vi "cal_inst.vi"() -> ()   [LabVIEW 2011]
panel:
  in  "Duration (0.00 seconds)":dbl format="%.2g"
  in  "Start Voltage (0.00 volts)":dbl format="%.2f"
  in  "End Voltage (0.00 volts)":dbl format="%.2g"
  out "Ramp In Progress":bool
  in  "Abort Ramp":bool
  in  "Current Limit (10.00 Amps)":dbl=10.0 format="%.2f"
  in  "Voltage Level (100.00 volts)":dbl=100.0 format="%.2f"
  in  "Voltage Range (150.00 volts)":dbl=150.0 format="%.2f"
  in  "Phase Name (\"\")":string
  in  "Frequency (60.00 Hz)":dbl=60.0 format="%.2f"
  in  "Frequency Range (600.00 Hz)":dbl=600.0 format="%.2f"
  in  "IVI Logical Name":refnum<k15>
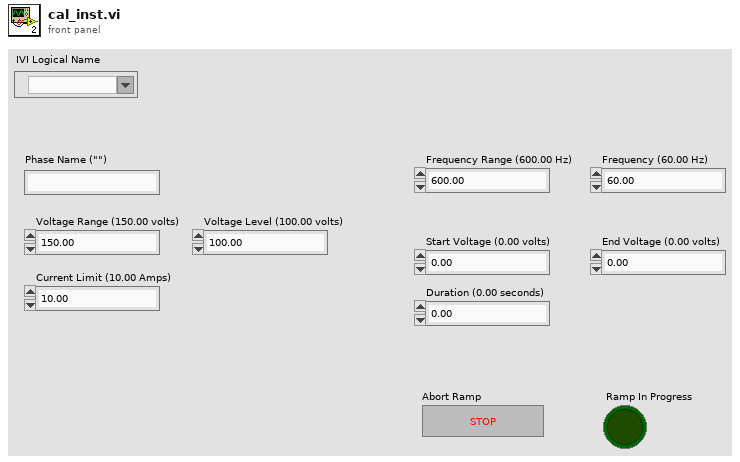
[diagram p1: front panel]
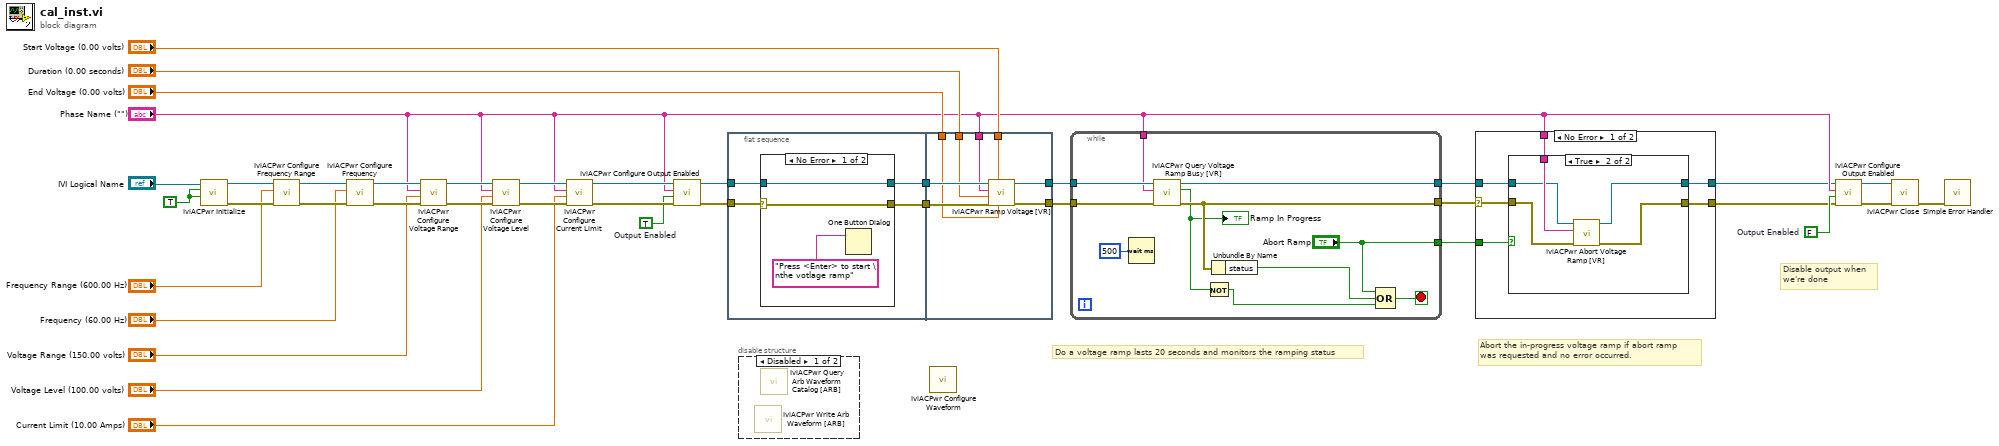
[diagram p0: block diagram]
diagram:
  w12 = FALSE  # Output Enabled
  w20 = TRUE  # Output Enabled
  w30 = TRUE ("id query (Yes)")
  # "Abort the in-progress voltage ramp if abort ramp\nwas requested and no error occurred."
  # "Disable output when\nwe're done"
  # "Do a voltage ramp lasts 20 seconds and monitors the ramping status"
  n1 = call <vilib>:"IviACPwr Initialize.vi"("reset device (Yes)"=w30, "id query (Yes)"=w30, "logical name (\"SampleACPwr\")"="IVI Logical Name") -> ("error out"=w36:errorcluster, "instrument handle out"=w37:refnum<k15>)  [unwired: 1 in, 6 out]
  n2 = call <vilib>:"IviACPwr Configure Frequency Range.vi"("error in (no error)"=w36, "Frequency Range"="Frequency Range (600.00 Hz)", "instrument handle"=w37) -> ("error out"=w34:errorcluster, "instrument handle out"=w35:refnum<k15>)  [unwired: 1 in, 6 out]
  n3 = call <vilib>:"IviACPwr Configure Frequency.vi"("error in (no error)"=w34, "Frequency"="Frequency (60.00 Hz)", "instrument handle"=w35) -> ("error out"=w32:errorcluster, "instrument handle out"=w33:refnum<k15>)  [unwired: 1 in, 6 out]
  n4 = call <vilib>:"IviACPwr Configure Voltage Range.vi"("error in (no error)"=w32, "Range"="Voltage Range (150.00 volts)", "Phase Name (\"\")"="Phase Name (\"\")", "instrument handle"=w33) -> ("error out"=w25:errorcluster, "instrument handle out"=w28:refnum<k15>)  [unwired: 6 out]
  n5 = call <vilib>:"IviACPwr Configure Voltage Level.vi"("error in (no error)"=w25, "Voltage Level"="Voltage Level (100.00 volts)", "Phase Name (\"\")"="Phase Name (\"\")", "instrument handle"=w28) -> ("error out"=w26:errorcluster, "instrument handle out"=w27:refnum<k15>)  [unwired: 6 out]
  n6 = call <vilib>:"IviACPwr Configure Current Limit.vi"("error in (no error)"=w26, "Limit"="Current Limit (10.00 Amps)", "Phase Name (\"\")"="Phase Name (\"\")", "instrument handle"=w27) -> ("error out"=w21:errorcluster, "instrument handle out"=w22:refnum<k15>)  [unwired: 6 out]
  n7 = call <vilib>:"IviACPwr Configure Output Enabled.vi"("error in (no error)"=w21, "Output Enabled (False)"=w20, "Phase Name (\"\")"="Phase Name (\"\")", "instrument handle"=w22) -> ("error out"=w17:errorcluster, "instrument handle out"=w18:refnum<k15>)  [unwired: 6 out]
  n8 = flat-sequence {
    tunnel: w18 -> [w43]
    tunnel: w17 -> [w42]
    tunnel: [w41] -> w39
    tunnel: [w40] -> w38
    tunnel: w39 -> [w56]
    tunnel: w38 -> [w55]
    tunnel: "Phase Name (\"\")" -> [w54]
    tunnel: [w53] -> w16
    tunnel: [w52] -> w15
    tunnel: "Duration (0.00 seconds)" -> [w51]
    tunnel: "Start Voltage (0.00 volts)" -> [w50]
    tunnel: "End Voltage (0.00 volts)" -> [w49]
    frame #0 {
      n9 = case shown="No Error" w42 {
        selector: w42 -> [w44 w47]
        tunnel: w43 -> [w45 w48]
        tunnel: [w45 w48] -> w41
        tunnel: [w44 w47] -> w40
        frame No Error {
          n10 = One Button Dialog(message="Press <Enter> to start \nthe votlage ramp") -> ()  [unwired: 2 out]
        }
        frame Error {
        }
      }
    }
    frame #1 {
      n11 = call <vilib>:"IviACPwr Ramp Voltage [VR].vi"("End Voltage"=w49, "Start Voltage"=w50, "error in (no error)"=w55, "Duration"=w51, "Phase Name (\"\")"=w54, "instrument handle"=w56) -> ("error out"=w52:errorcluster, "instrument handle out"=w53:refnum<k15>)  [unwired: 4 out]
    }
  }
  n12 = disable-structure shown="Disabled" {
    frame Disabled {
      n13 = call <vilib>:"IviACPwr Write Arb Waveform [ARB].vi"() -> ()  [unwired: 10 in, 2 out]
      n14 = call <vilib>:"IviACPwr Query Arb Waveform Catalog [ARB].vi"() -> ()  [unwired: 9 in, 3 out]
    }
    frame Enabled {
    }
  }
  n15 = call <vilib>:"IviACPwr Configure Waveform.vi"() -> ()  [unwired: 10 in, 2 out]
  n16 = while {
    tunnel: w16 -> [w67]
    tunnel: w15 -> [w66]
    tunnel: [w65] -> w4
    tunnel: [w64] -> w6
    tunnel: "Phase Name (\"\")" -> [w59]
    tunnel: ["Abort Ramp"] -> w5
    stop <- w62 stop-if-true
    n17 = Wait (ms)(milliseconds to wait=u32 500) -> ()  [unwired: 1 out]
    n18 = call <vilib>:"IviACPwr Query Voltage Ramp Busy [VR].vi"("error in (no error)"=w66, "Phase Name (\"\")"=w59, "instrument handle"=w67) -> ("error out"=w64:errorcluster, "Busy"=w63:bool, "instrument handle out"=w65:refnum<k15>)  [unwired: 6 out]
    "Ramp In Progress" <- w63
    n19 = Not(x=w63) -> (.not. x?=w61:bool)
    n20 = Unbundle By Name(w64) -> ("status"=w58:bool)
    n21 = Compound Arithmetic op=OR("Abort Ramp", w58, w61) -> (w62:bool)
  }
  n22 = case shown="No Error" w6 {
    selector: w6 -> [w71 w81]
    tunnel: w5 -> [w73 _]
    tunnel: w4 -> [w72 w82]
    tunnel: "Phase Name (\"\")" -> [w70 _]
    tunnel: [w69 w82] -> w2
    tunnel: [w68 w81] -> w1
    frame No Error {
      n23 = case shown="True" w73 {
        tunnel: w72 -> [w75 w79]
        tunnel: w71 -> [w74 w78]
        tunnel: w70 -> [_ w80]
        tunnel: [w75 w77] -> w69
        tunnel: [w74 w76] -> w68
        frame False {
        }
        frame True {
          n24 = call <vilib>:"IviACPwr Abort Voltage Ramp [VR].vi"("error in (no error)"=w78, "Phase Name (\"\")"=w80, "instrument handle"=w79) -> ("error out"=w76:errorcluster, "instrument handle out"=w77:refnum<k15>)  [unwired: 7 out]
        }
      }
    }
    frame Error {
    }
  }
  n25 = call <vilib>:"IviACPwr Configure Output Enabled.vi"("error in (no error)"=w1, "Output Enabled (False)"=w12, "Phase Name (\"\")"="Phase Name (\"\")", "instrument handle"=w2) -> ("error out"=w14:errorcluster, "instrument handle out"=w13:refnum<k15>)  [unwired: 6 out]
  n26 = call <vilib>:"IviACPwr Close.vi"("error in (no error)"=w14, "instrument handle"=w13) -> ("error out"=w19:errorcluster)  [unwired: 9 out]
  n27 = call <vilib>:"Simple Error Handler.vi"("error in (no error)"=w19) -> ()  [unwired: 1 in, 8 out]
